vi "VoltajeDeseado.vi"(8 "error in (no error)":errorcluster, 9 "Nivel Medido (dB)":dbl=1000.0 format="%#_13g", 10 "Nivel Emitido (dB)":dbl=1000.0 format="%#_13g") -> (0 "error out":errorcluster, 2 "Vdeseado":dbl, 3 "AjustesPrevios out":refnum<class "AjustesPrevios.lvclass">)   [LabVIEW 2019, in "AjustesPrevios.lvclass"]
uses:
  AjustesPrevios.lvclass
  Instrumento/Keithley2002/Keithley2002.lvclass
panel:
  out "VAC":string
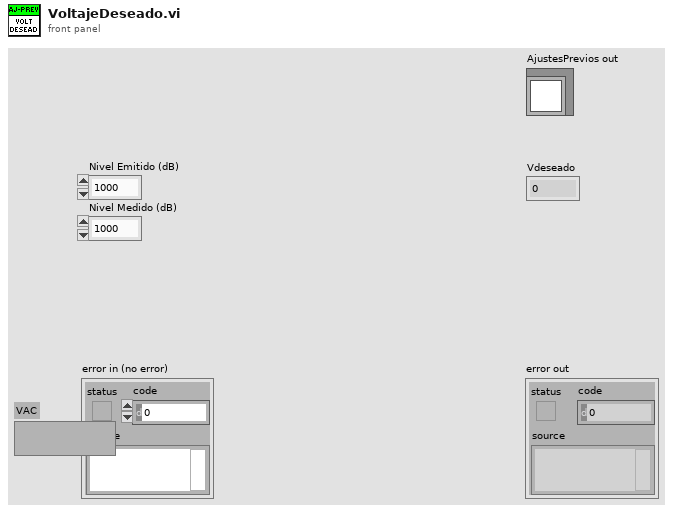
[diagram p1: front panel]
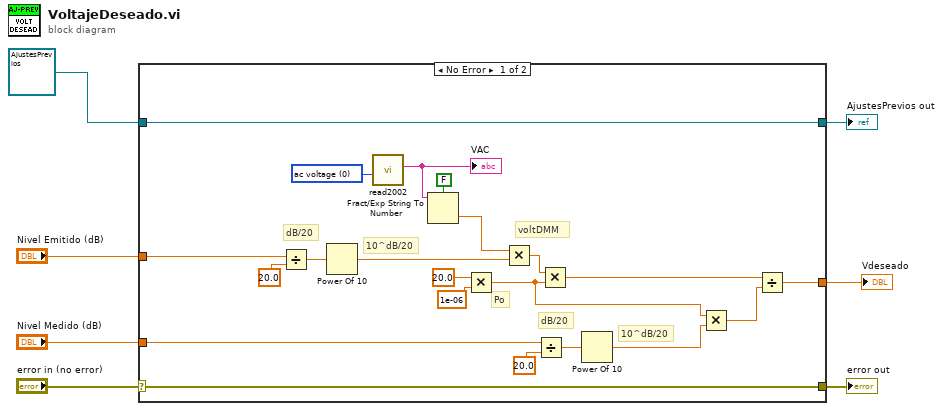
[diagram p0: block diagram]
diagram:
  n1 = case shown="No Error" "error in (no error)" {
    selector: "error in (no error)" -> [w27 w30]
    tunnel: [w27 w30] -> w6
    tunnel: [w28 w29] -> w4
    tunnel: refnum<class "AjustesPrevios.lvclass"> refnum ("AjustesPrevios in") -> [w28 w29]
    tunnel: "Nivel Emitido (dB)" -> [w20 _]
    tunnel: "Nivel Medido (dB)" -> [w13 _]
    tunnel: [w8 _] -> w1
    frame No Error {
      w26 = u16 0 items=["ac voltage", "dc voltage", "2-wire resistance", "4-wire resistance", "ac current", "dc current", "frequency", "temperature"] ("function (Vdc:1)")
      # "10^dB/20"
      # "dB/20"
      # "voltDMM"
      # "10^dB/20"
      # "dB/20"
      # "Po"
      n2 = Divide(x=w20, y=20.0 ("x")) -> (x/y=w18:dbl)
      n3 = Power Of 10(x=w18) -> (10^x=w17:dbl)
      n4 = call "read2002.vi"("function (Vdc:1)"=w26) -> ("Reading Result"=w24:string)  [unwired: 7 in, 3 out]
      "VAC" <- w24
      n5 = Fract/Exp String To Number(use system decimal point (T)=FALSE, string=w24) -> (number=w21:dbl)  [unwired: 2 in, 1 out]
      n6 = Multiply(x=20.0, y=1e-06) -> (x*y=w11:dbl)
      n7 = Multiply(x=w21, y=w17) -> (x*y=w16:dbl)
      n8 = Divide(x=w13, y=20.0 ("x")) -> (x/y=w15:dbl)
      n9 = Multiply(x=w16, y=w11) -> (x*y=w10:dbl)
      n10 = Power Of 10(x=w15) -> (10^x=w12:dbl)
      n11 = Multiply(x=w11, y=w12) -> (x*y=w9:dbl)
      n12 = Divide(x=w10, y=w9) -> (x/y=w8:dbl)
    }
    frame Error {
    }
  }
  "error out" <- w6
  "AjustesPrevios out" <- w4
  "Vdeseado" <- w1
